vi "UART Get Bytes Available.vi"(8 "Error In":errorcluster, 10 "UART Channel (0)":u8, 11 "LINX Resource":T1) -> (0 "Error Out":errorcluster, 1 "Bytes Available":u32, 3 "LINX Resource":T1)   [LabVIEW 2011, in "LVH-LINX.lvlib"]
doc: "Get the number of bytes available in the specified UART channel's receive buffer."
uses:
  LVH-LINX.lvlib
  Private/Type Defs/LINX Ref.ctl
  Private/Type Defs/Platform.ctl
  Private/Type Defs/Interface.ctl
  Private/Device/Type Defs/LINX Device Config.ctl
  Private/Device/Type Defs/TCP Config.ctl
  Private/Device/Type Defs/Channels.ctl
  Private/Type Defs/Peripheral.ctl
  Private/Type Defs/Channel FGV States.ctl
  Private/Device/Device.lvlib
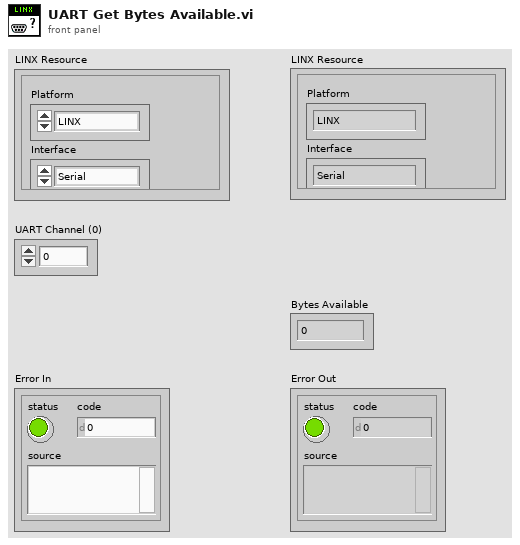
[diagram p1: front panel]
types:
  T1 = typedef "LVH-LINX.lvlib/LINX Ref.ctl" = cluster{"Platform":T2, "Interface":T3, "LINX Device Config":T4}
  T2 = typedef "LVH-LINX.lvlib/Platform.ctl" = enum16{"LINX", "myRIO"}
  T3 = typedef "LVH-LINX.lvlib/Interface.ctl" = enum16{"Serial", "TCP"}
  T4 = typedef "LVH-LINX.lvlib/Device.lvlib/LINX Device Config.ctl" = cluster{"Interface":T3, "COM Port":refnum<visa-resource-name>, "TCP Configuration":T5, "Device Family":u8, "Device ID":u8, "Device Name":string, "TCP Ref":refnum<k5>, "Channels":T6}
  T5 = typedef "LVH-LINX.lvlib/Device.lvlib/TCP Config.ctl" = cluster{"IP Address":string, "Port":u16}
  T6 = typedef "LVH-LINX.lvlib/Channels.ctl" = cluster{"DI Channels":u8[], "DO Channels":u8[], "AI":u8[], "AO":u8[], "PWM":u8[], "QE":u8[], "UART":u8[], "I2C 2":u8[], "SPI":u8[], "CAN":u8[], "AI Ref (V)":dbl, "AO Resolution (Bits)":u8, "AO Ref (V)":dbl}
  T7 = typedef "LVH-LINX.lvlib/Peripheral.ctl" = enum8{"DI", "DO", "AI", "AO", "PWM", "QE", "UART", "I2C", "SPI", "CAN"}
  T8 = typedef "LVH-LINX.lvlib/Channel FGV States.ctl" = enum16{"Initialize", "Get", "Set"}
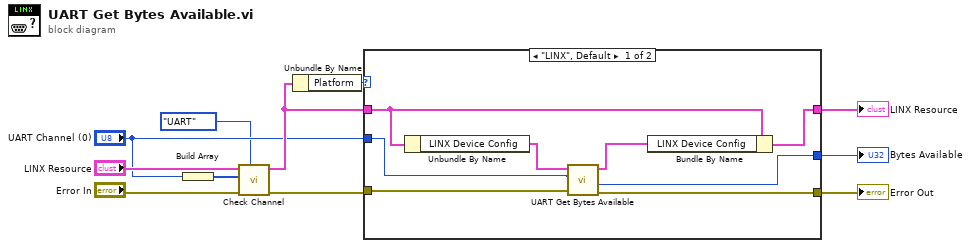
[diagram p0: block diagram]
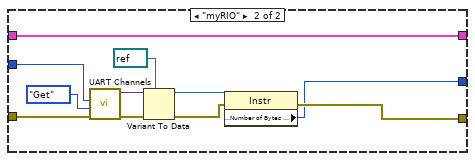
[diagram p2: hidden frame]
diagram:
  n1 = Build Array("UART Channel (0)") -> (w4:u8[])
  n2 = call "Check Channel.vi"("Peripheral"=Peripheral."UART", "Error In"="Error In", "Channels"=w4, "LINX Resource"="LINX Resource") -> ("Error Out"=w5:errorcluster, "LINX Resource"=w6:T1)  [unwired: 5 in, 1 out]
  n3 = Unbundle By Name(w6) -> ("Platform"=w11:T2)
  n4 = case shown="\"LINX\", Default" w11 {
    tunnel: w5 -> [w16 w29]
    tunnel: w6 -> [w19 w30]
    tunnel: [w17 w21] -> w10
    tunnel: [w18 w30] -> w9
    tunnel: "UART Channel (0)" -> [w15 w23]
    tunnel: [w12 w20] -> w1
    frame "LINX", Default {
      n5 = Unbundle By Name(w19) -> ("LINX Device Config"=w14:T4)
      n6 = call "UART Get Bytes Available.vi"("Error In"=w16, "UART Channel"=w15, "LINX Device Config"=w14) -> ("Error Out"=w17:errorcluster, "Bytes Availabe"=w12:u8, "LINX Device Config"=w13:T4)  [unwired: 6 in]
      n7 = Bundle By Name(cluster=w19, "LINX Device Config"=w13) -> (w18:T1)
    }
    frame "myRIO" {
      n8 = call "UART Channels.vi"("Error In"=w29, "Channel State"=Channel_FGV_States."Get", "Channel Number"=w23) -> ("Error Out"=w28:errorcluster, "UART Channel"=w27:variant)  [unwired: 7 in]
      n9 = Variant To Data(error in=w28, type=refnum<visa-resource-name> refnum ("reference"), Variant=w27) -> (data=w25:refnum<visa-resource-name>, error out=w24:errorcluster)
      n10 = property class="Instr"(reference=w25, error in=w24) -> (error out=w21:errorcluster, "Serial Settings:Number of Bytes at Serial Port"=w20:u32)  [unwired: 1 out]
    }
  }
  "Error Out" <- w10
  "LINX Resource" <- w9
  "Bytes Available" <- w1
